vi "BeamformerTop.vi"() -> ()   [LabVIEW 2013]
uses:
  <vilib>/express/express analysis/Spectral/Block/exnSpectralBlock spectral measurements RMS poly.vi
  <vilib>/express/express analysis/Spectral/Block/exnSpectralBlock spectral measurements RMS WFM.vi
  <vilib>/express/express analysis/Spectral/XNode/ExpressSpectralMeasurementsBlockNode.xnode
panel:
  out "Beamformer Output 2":cluster{"f0":dbl, "df":dbl, "magnitude":dbl[]}(graph)
  out "Microphone Input 2":cluster{"f0":dbl, "df":dbl, "magnitude":dbl[]}(graph)
  out "Beamformer Output":waveform(dbl)(graph)
  out "Microphone Input":dynamicdata(graph)
  in  "stop (F)":bool
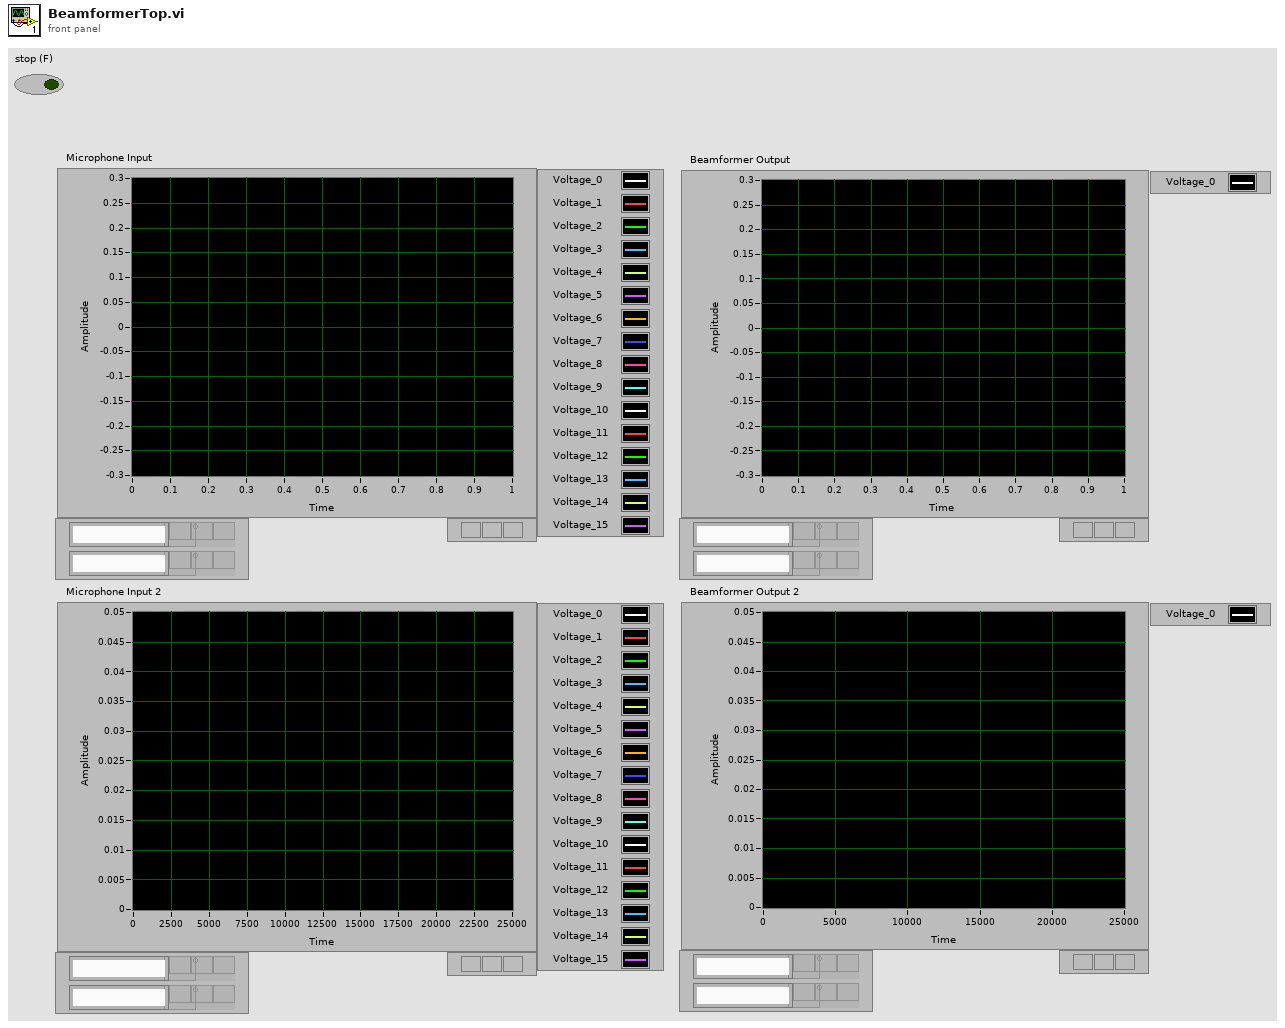
[diagram p1: front panel]
types:
  T1 = cluster{"averaging mode":u16, "weighting mode":u16, "number of averages":u32}
  T2 = cluster{"dB On (F)":bool, "unwrap phase (F)":bool, "convert to degree (F)":bool}
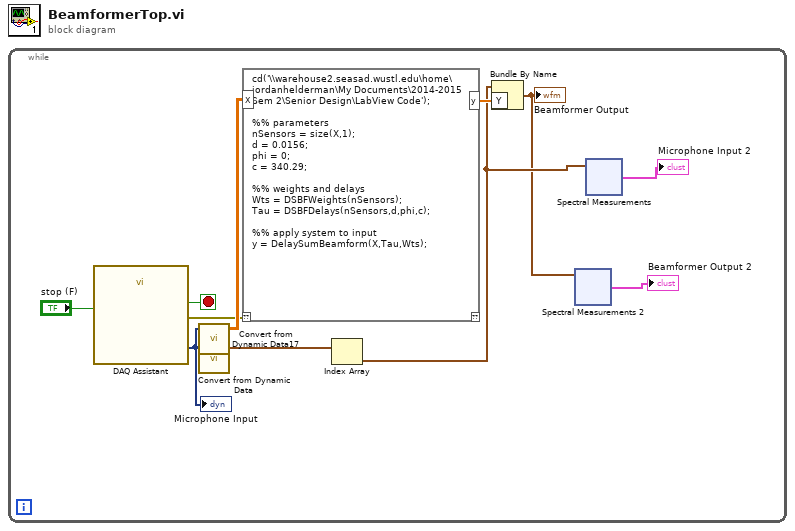
[diagram p0: block diagram]
diagram:
  n1 = while {
    stop <- w10 stop-if-true
    n2 = call "DAQ Assistant"("stop (F)"="stop (F)") -> ("data"=w8:dynamicdata, "stopped"=w10:bool, "error out"=w6:errorcluster)  [unwired: 15 in, 1 out]
    "Microphone Input" <- w8
    n3 = call "Convert from Dynamic Data17"("Dynamic Data Type"=w8) -> ("Array"=w9:dbl[][])  [unwired: 3 in]
    n4 = call "Convert from Dynamic Data"("Dynamic Data Type"=w8) -> ("Array of Waveform"=w7:waveform(dbl)[])  [unwired: 3 in]
    n5 = script code="cd('\\\\warehouse2.seasad.wustl.edu\\home\\jordanhelderman\\My Documents\\2014-2015 Sem 2\\Senior Design\\LabView Code');\n\n%% parameters\nnSensors = size(X,1);\nd = 0.0156;\nphi = 0;\nc = 340.29;\n\n%% weights and delays\nWts = DSBFWeights(nSensors);\nTau = DSBFDelays(nSensors,d,phi,c);\n\n%% apply system to input\ny = DelaySumBeamform(X,Tau,Wts);"("??"=w6, "X"=w9) -> ("y"=w5:dbl[])  [unwired: 1 out]
    n6 = Index Array(array=w7) -> (element=w4:waveform(dbl))  [unwired: 1 in]
    n7 = Bundle By Name(cluster=w4, "Y"=w5) -> (w3:waveform(dbl))
    "Beamformer Output" <- w3
    n8 = xnode "Spectral Measurements 2"("Signals"=w3) -> ("FFT - (RMS)"=→"Beamformer Output 2":cluster{"f0":dbl, "df":dbl, "magnitude":dbl[]})  [unwired: 1 in, 2 out]
    n9 = xnode "Spectral Measurements"("Signals"=w4) -> ("FFT - (RMS)"=→"Microphone Input 2":cluster{"f0":dbl, "df":dbl, "magnitude":dbl[]})  [unwired: 1 in, 2 out]
  }
